vi "CMI ADS127L21 - Config Virtual Channels.vi"(8 "error in (no error)":errorcluster, 11 "ADS127L21 session":T1 {"channels"."Channel" min=1 max=8 step=1}) -> (0 "error out":errorcluster, 1 "virtual channel idns":string[](array[string]), 2 "idn string":string, 3 "ADS127L21 session out":T1 {"channels"."Channel" min=1 max=8 step=1})   [LabVIEW 2020]
uses:
  CMI ADS127L21 - Input Range.ctl
  CMI ADS127L21 - Input Mode.ctl
  CMI ADS127L21 - Input Impedance.ctl
  CMI ADS127L21 - Record Channel.ctl
  CMI ADS127L21 - EXTOUT Mode.ctl
  CMI ADS127L21 - EXTOUT Polarity.ctl
  CMI ADS127L21 - Session.ctl
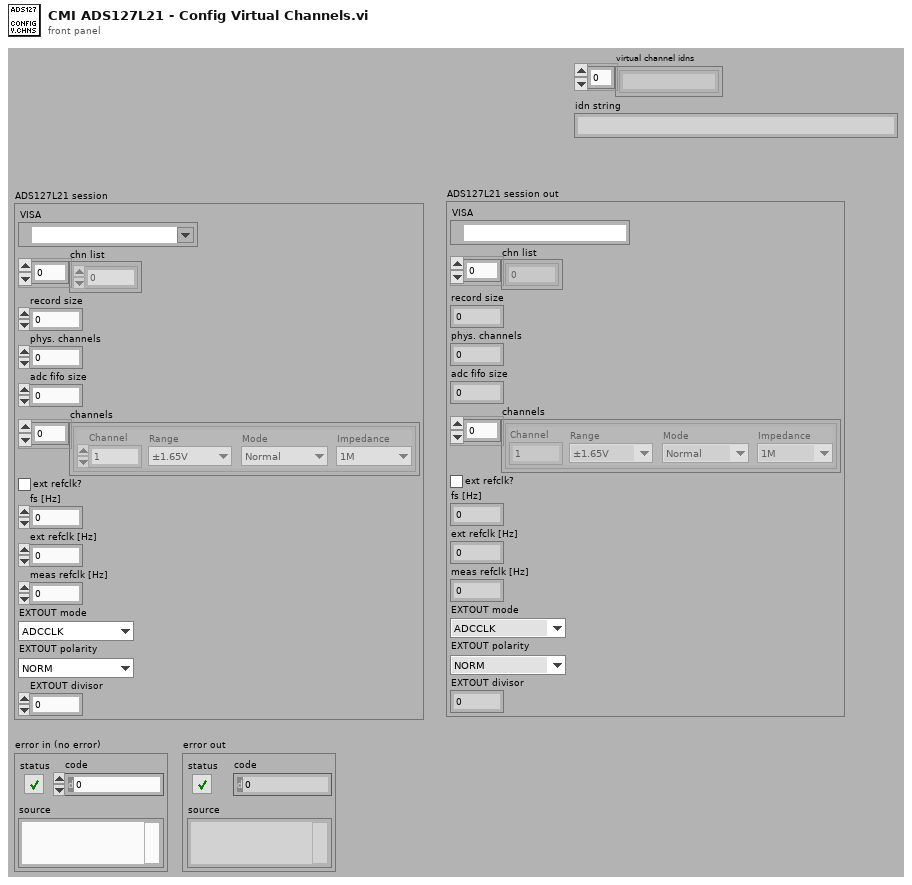
[diagram p1: front panel]
types:
  T1 = typedef "CMI ADS127L21 - Session.ctl" = cluster{"VISA":refnum<visa-resource-name>, "chn list":i32[], "record size":i32, "phys. channels":i32, "adc fifo size":i32, "channels":T2[], "ext refclk?":bool, "fs [Hz]":dbl, "ext refclk [Hz]":dbl, "meas refclk [Hz]":dbl, "EXTOUT mode":T6, "EXTOUT polarity":T7, "EXTOUT divisor":i32}
  T2 = typedef "CMI ADS127L21 - Record Channel.ctl" = cluster{"Range":T3, "Channel":i32, "Mode":T4, "Impedance":T5}
  T3 = typedef "CMI ADS127L21 - Input Range.ctl" = enum16{"±1.65V", "±2V"}
  T4 = typedef "CMI ADS127L21 - Input Mode.ctl" = enum16{"Normal", "Inverted", "GND"}
  T5 = typedef "CMI ADS127L21 - Input Impedance.ctl" = enum16{"1M", "1k5"}
  T6 = typedef "CMI ADS127L21 - EXTOUT Mode.ctl" = enum16{"ADCCLK", "REFCLK", "SMPLCLK", "FIRST"}
  T7 = typedef "CMI ADS127L21 - EXTOUT Polarity.ctl" = enum16{"NORM", "INV"}
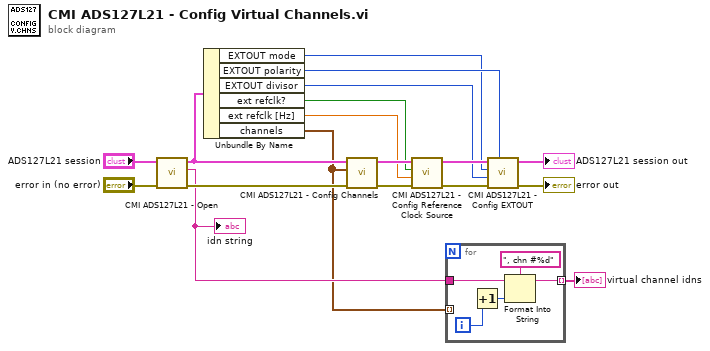
[diagram p0: block diagram]
diagram:
  n1 = call "CMI ADS127L21 - Open.vi"("error in (no error)"="error in (no error)", "session in"="ADS127L21 session") -> ("error out"=w16:errorcluster, "idn string"=w3:string, "session out"=w15:T1)  [unwired: 7 in]
  "idn string" <- w3
  n2 = Unbundle By Name(w15) -> ("EXTOUT mode"=w7:T6, "EXTOUT polarity"=w8:T7, "EXTOUT divisor"=w6:i32, "ext refclk?"=w12:bool, "ext refclk [Hz]"=w11:dbl, "channels"=w2:T2[])
  n3 = call "CMI ADS127L21 - Config Channels.vi"("error in (no error)"=w16, "Channels"=w2, "session in"=w15) -> ("error out"=w14:errorcluster, "session out"=w13:T1)  [unwired: 7 in]
  n4 = call "CMI ADS127L21 - Config Reference Clock Source.vi"("error in (no error)"=w14, "External Refclk Freq [Hz]"=w11, "Use External Source? (False: Internal)"=w12, "session in"=w13) -> ("error out"=w10:errorcluster, "session out"=w9:T1)  [unwired: 6 in]
  n5 = for {
    tunnel: w3 -> [w22]
    tunnel: [w21] -> w1 mode=indexing
    tunnel: w2 -> [_] mode=indexing
    i -> [w19]
    n6 = Increment(x=w19) -> (x+1=w20:i32)
    n7 = Format Into String(format string=", chn #%d", initial string=w22, w20) -> (resulting string=w21:string)  [unwired: 1 in, 1 out]
  }
  "virtual channel idns" <- w1
  n8 = call "CMI ADS127L21 - Config EXTOUT.vi"("Polarity"=w8, "error in (no error)"=w10, "Divisor (1)"=w6, "Mode"=w7, "session in"=w9) -> ("error out"=→"error out":errorcluster, "session out"=→"ADS127L21 session out":T1)  [unwired: 5 in]
